vi "Auto Path Names.vi"() -> (3 "Path Names":string[](array[string]))   [LabVIEW 2019]
uses:
  <vilib>/Rock Robotics/Network Tables/NT Read String.vi
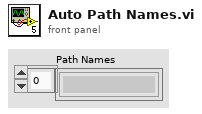
[diagram p1: front panel]
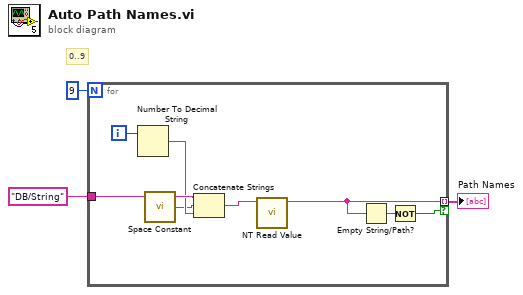
[diagram p0: block diagram]
diagram:
  # "0..9"
  n1 = for {
    N: 9 -> [_]
    tunnel: "DB/String" -> [w11]
    tunnel: [w9] -> w1 mode=indexing if=w7
    i -> [w6]
    n2 = Number To Decimal String(number=w6) -> (decimal integer string=w5:string)  [unwired: 1 in]
    n3 = call <vilib>:"Space Constant.vi"() -> ("String"=w4:string)
    n4 = Concatenate Strings(w11, w4, w5) -> (w10:string)
    n5 = call-poly <vilib>:"NT Read Value.vi"("Name"=w10) -> ("String"=w9:string)  [unwired: 9 in, 1 out]
    n6 = Empty String/Path?(string/path=w9) -> (empty?=w8:bool)
    n7 = Not(x=w8) -> (.not. x?=w7:bool)
  }
  "Path Names" <- w1
